vi "Test 7z.bat.vi"() -> ()   [LabVIEW 2016, in "PostBuildSupport.lvclass"]
uses:
  PostBuildSupport.lvclass
  PostBuildSupport.lvclass/PostBuildSupport.ctl
panel:
  in  "Product Name":string
  in  "Package Source Folder":path
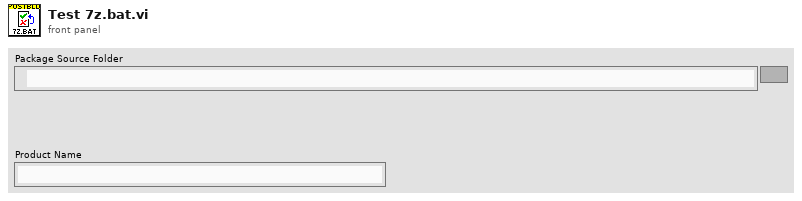
[diagram p1: front panel]
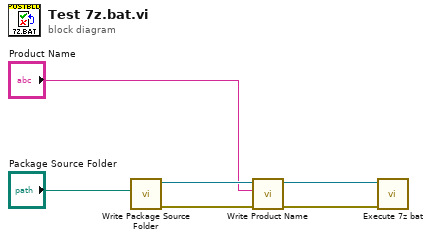
[diagram p0: block diagram]
diagram:
  n1 = call "Write Package Source Folder.vi"("Package Source Folder"="Package Source Folder") -> ("error out"=w5:errorcluster, "PostBuildSupport out"=w6:refnum<class "PostBuildSupport.lvclass">)  [unwired: 9 in]
  n2 = call "Write Product Name.vi"("error in (no error)"=w5, "Product Name"="Product Name", "PostBuildSupport in"=w6) -> ("error out"=w3:errorcluster, "PostBuildSupport out"=w4:refnum<class "PostBuildSupport.lvclass">)  [unwired: 7 in]
  n3 = call "Execute 7z bat.vi"("error in (no error)"=w3, "PostBuildSupport in"=w4) -> ()  [unwired: 8 in, 2 out]
